vi "Svg Creat Color.vi"(8 "error in (no error)":errorcluster, 10 "color":u32(colorbox)=141) -> (0 "error out":errorcluster, 3 ".NET Refnum out":refnum<k24>)   [LabVIEW 2020, in "SvgDotNet.lvlib"]
uses:
  SvgDotNet.lvlib
  C:/Users/huipeng8/Desktop/SVG.NET/Svg.dll
  Svg.dll
  System.Drawing
panel:
  # "Connector Pane"
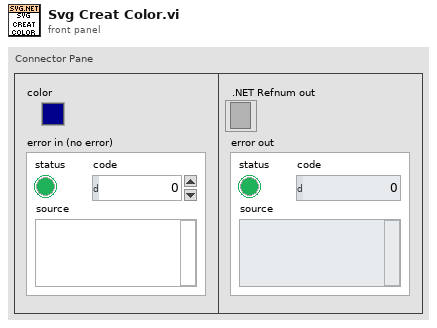
[diagram p1: front panel]
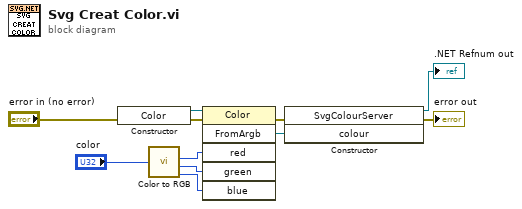
[diagram p0: block diagram]
diagram:
  n1 = constructor class="Color"(error in="error in (no error)") -> (reference out=w7:refnum<k24>, error out=w8:errorcluster)  [unwired: 2 in, 1 out]
  n2 = call <vilib>:"Color to RGB.vi"("Color"="color") -> ("R"=w4:u8, "G"=w3:u8, "B"=w2:u8)  [unwired: 1 out]
  n3 = invoke class="Color" method="FromArgb"(reference=w7, error in=w8, "red"=w4, "green"=w3, "blue"=w2) -> (error out=w9:errorcluster, "FromArgb"=w5:refnum<k24>)  [unwired: 1 in, 4 out]
  n4 = constructor class="SvgColourServer"(error in=w9, "colour"=w5) -> (reference out=→".NET Refnum out":refnum<k24>, error out=→"error out":errorcluster)  [unwired: 2 in, 2 out]
